vi "subCloseConfigurationPageRefs.vi"(11 "References":T1) -> (0 "error out":errorcluster, 3 "Rule parser info.References":T1)   [LabVIEW 2020, in "UserInterface.lvlib" / "UIManager.lvclass"]
uses:
  UIManager.lvclass
  subReferenceData.ctl
  ExtensionInterfaces/IConfigurationPage/Event_Stop.ctl
  ExtensionInterfaces/IConfigurationPage/Event_Parameters.ctl
  d5166041-e29f-4ca9-83be-f4ffdef9043e.vi
  ExtensionInterfaces/IConfigurationPage/IConfigurationPage.lvclass
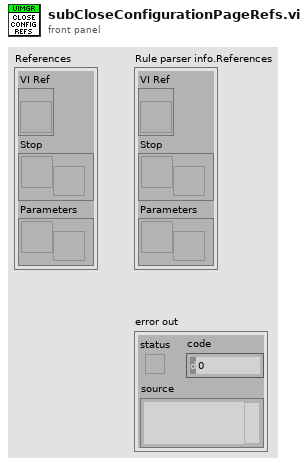
[diagram p1: front panel]
types:
  T1 = typedef "UserInterface.lvlib/UIManager.lvclass/subReferenceData.ctl" = cluster{"VI Ref":refnum<vi>, "Stop":refnum<user-event>, "Parameters":refnum<user-event>}
  T2 = typedef "ExtensionInterfaces.lvlib/IConfigurationPage.lvclass/Event_Stop.ctl" = cluster{"Stop":bool}
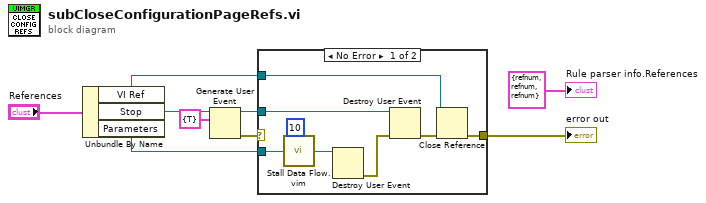
[diagram p0: block diagram]
diagram:
  n1 = Unbundle By Name("References") -> ("VI Ref"=w1:refnum<vi>, "Stop"=w4:refnum<user-event>, "Parameters"=w2:refnum<user-event>)
  n2 = Generate User Event(user event=w4, event data cluster=T2 {"Stop"=TRUE} ("event data")) -> (user event out=w5:refnum<user-event>, error out=w6:errorcluster)  [unwired: 2 in]
  n3 = case shown="No Error" w6 {
    tunnel: w1 -> [w17 _]
    tunnel: w2 -> [w11 _]
    tunnel: [w13 _] -> w7
    tunnel: w5 -> [w16 _]
    frame No Error {
      n4 = call "Stall Data Flow.vim"("value in"=w11, "milliseconds to wait"=u32 10) -> ("value out"=w12:refnum<user-event>)  [unwired: 1 out]
      n5 = Destroy User Event(user event=w12) -> (error out=w15:errorcluster)  [unwired: 1 in]
      n6 = Destroy User Event(user event=w16, error in=w15) -> (error out=w14:errorcluster)
      n7 = Close Reference(reference=w17, error in (no error)=w14) -> (error out=w13:errorcluster)
    }
    frame Error {
    }
  }
  "error out" <- w7
  "Rule parser info.References" <- T1 {"VI Ref"=refnum, "Stop"=refnum, "Parameters"=refnum} ("Rule parser info.References")
